vi "glADC.vi"() -> ()   [LabVIEW 2012]
panel:
  in  "ADC 7609":T1={"OS"=0, "Range"=1, "T_hi"=2, "D_low"=2} {"Range" items=["+-20V", "+-10V", "+-5V"]; "OS" items=["NONE", "2X", "4X", "8X", "16X", "32X", "64"]}
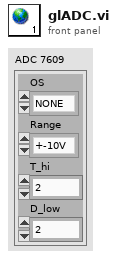
[diagram p1: front panel]
types:
  T1 = cluster{"OS":u8, "Range":u8, "T_hi":u8, "D_low":u8}
diagram:
